vi "get_number_frames.vi"(2 "error in":errorcluster, 3 "Trajectory (JSON)":string) -> (0 "error out":errorcluster, 1 "Number of frames":i32)   [LabVIEW 2019]
doc: "Obtain the number of trajectories on the Trajectory Configuration text."
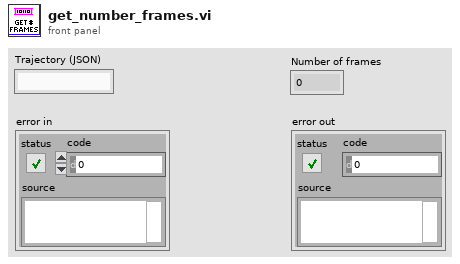
[diagram p1: front panel]
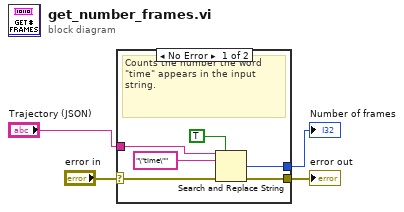
[diagram p0: block diagram]
diagram:
  n1 = case shown="No Error" "error in" {
    selector: "error in" -> [w8 w11]
    tunnel: [w7 w11] -> w3
    tunnel: [w6 _] -> w1
    tunnel: "Trajectory (JSON)" -> [w5 _]
    frame No Error {
      # "Counts the number the word \"time\" appears in the input string."
      n2 = Search and Replace String(replace all?=TRUE ("replace all? (F)"), input string=w5, search string="\"time\"", error in=w8) -> (number of replacements=w6:i32, error out=w7:errorcluster)  [unwired: 4 in, 2 out]
    }
    frame Error {
    }
  }
  "error out" <- w3
  "Number of frames" <- w1
